vi "Timing Message Loop.vi"(8 "error in (no error)":errorcluster, 10 "Timers":T1, 11 "Message Queues":T2) -> (0 "error out":errorcluster)   [LabVIEW 2017, in "Message Queue.lvlib"]
uses:
  Message Queue.lvlib
  All Message Queues.ctl
  Message Cluster.ctl
  Acquisition/Acquisition State.ctl
  11995cb8-e311-3fce-f8c0-29dfdff9c03f.vi
  controls/ExitGlobal.vi
  Enqueue Message (Single).vi
  <vilib>/Utility/error.llb/Error Cluster From Error Code.vi
  <vilib>/ErrorRing/Error Ring.xnode
  Acquisition/Acquisition.lvlib
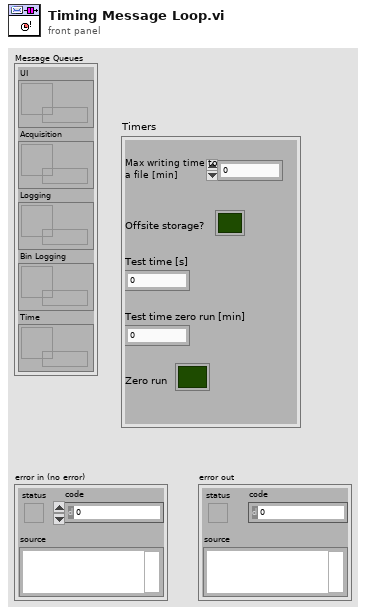
[diagram p1: front panel]
types:
  T1 = cluster{"Offsite storage?":bool, "Test time [s]":dbl, "Test time zero run [s] ":dbl, "Max writing time to a file [min]":dbl, "Zero run":bool}
  T2 = typedef "Message Queue.lvlib/All Message Queues.ctl" = cluster{"UI":refnum<queue>, "Acquisition":refnum<queue>, "Logging":refnum<queue>, "Bin Logging":refnum<queue>, "Time":refnum<queue>}
  T3 = typedef "Acquisition.lvlib/Acquisition State.ctl" = enum16{"Idle", "Acquiring"}
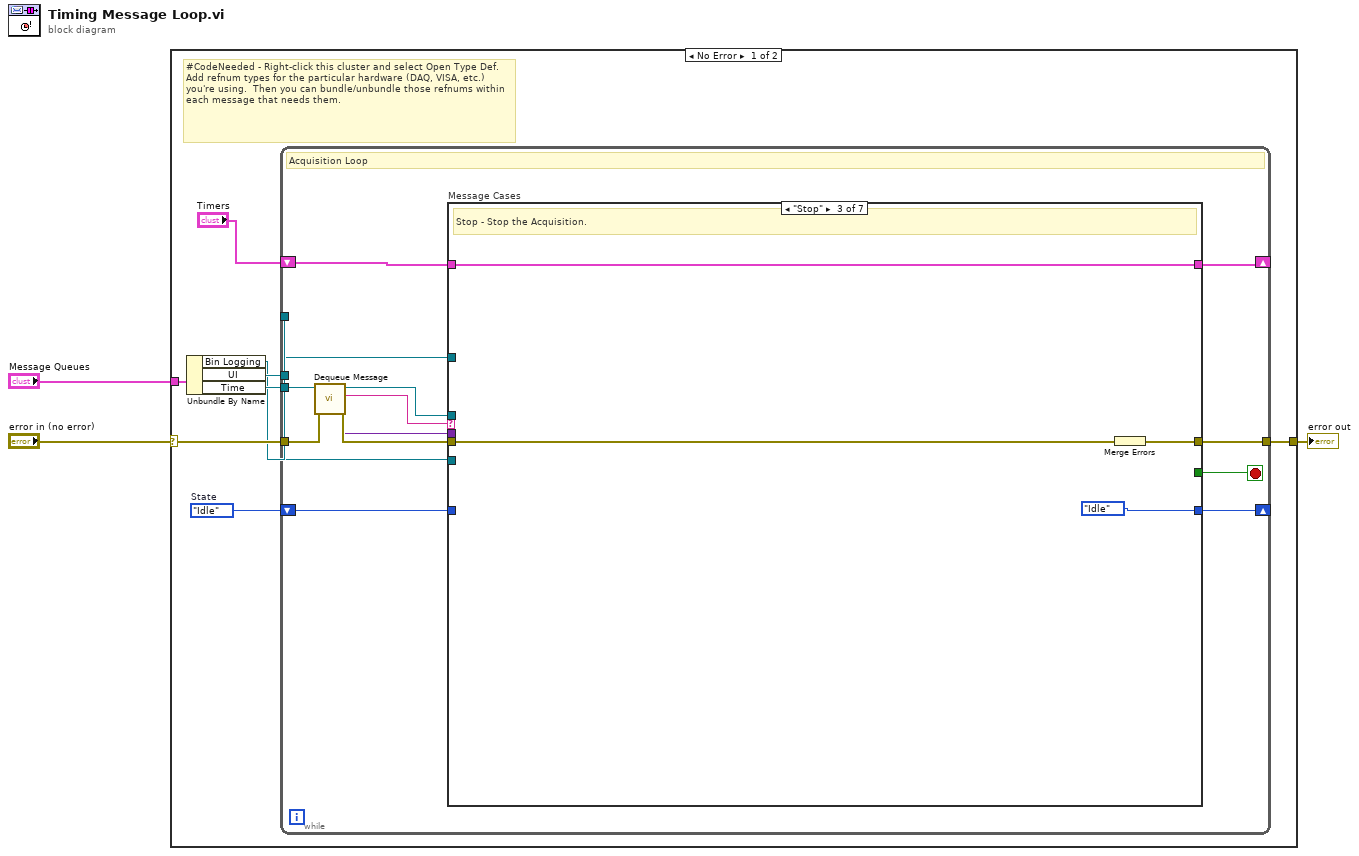
[diagram p0: block diagram]
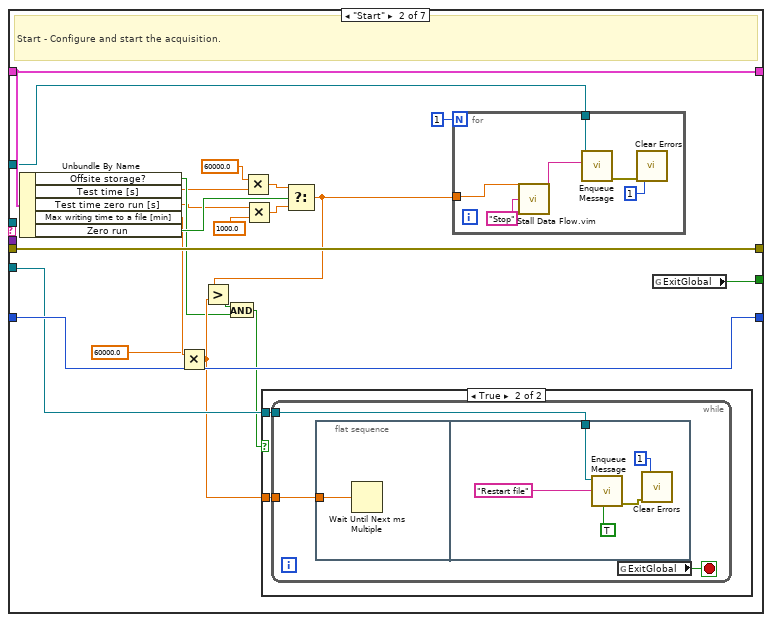
[diagram p3: hidden frame]
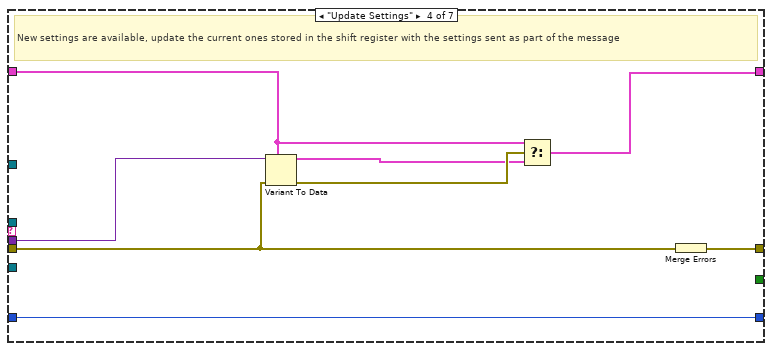
[diagram p5: hidden frame]
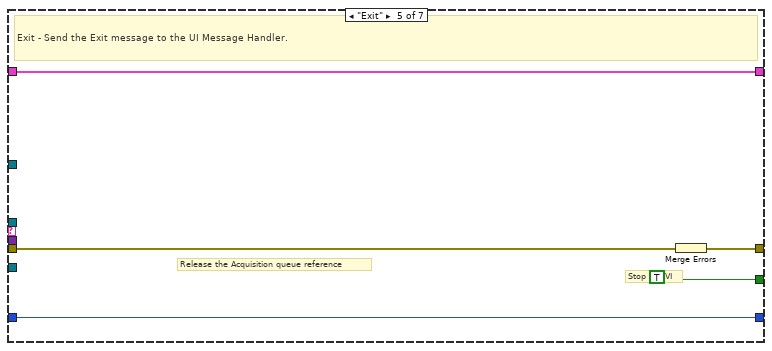
[diagram p6: hidden frame]
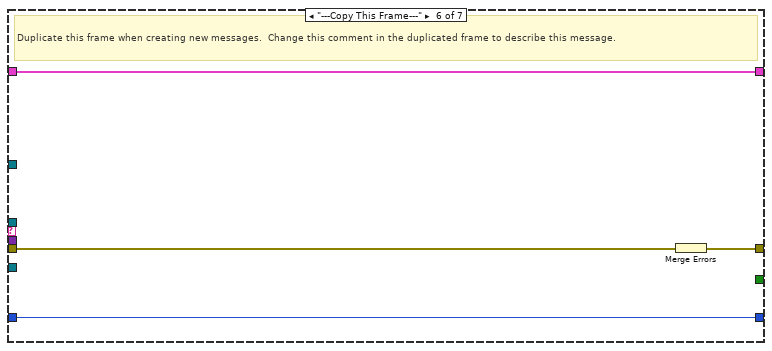
[diagram p7: hidden frame]
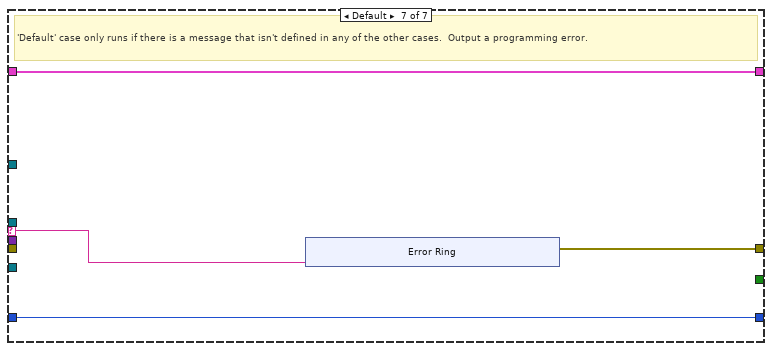
[diagram p8: hidden frame]
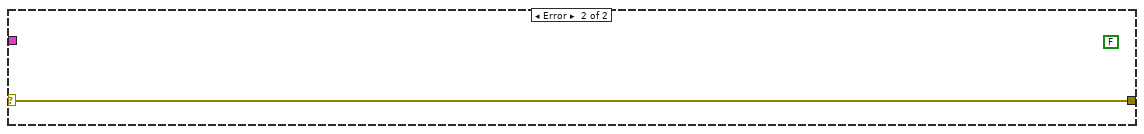
[diagram p9: hidden frame]
diagram:
  n1 = case shown="No Error" "error in (no error)" {
    selector: "error in (no error)" -> [w9 w99]
    tunnel: "Message Queues" -> [w11 _]
    tunnel: [w5 w99] -> w2
    frame No Error {
      w7 = Acquisition_State."Idle"  # State
      # "#CodeNeeded - Right-click this cluster and select Open Type Def.  Add refnum types for the particular hardware (DAQ, VISA, etc.) you're using.  Then you can bundle/unbundle those refnums within each message that needs them."
      n2 = Unbundle By Name(w11) -> ("Bin Logging"=w4:refnum<queue>, "UI"=w8:refnum<queue>, "Time"=w10:refnum<queue>)
      n3 = while {
        tunnel: w10 -> [w20]
        shift-right: [w24] -> _
        shift-left: "Timers" -> [w25]
        tunnel: w8 -> [w16]
        shift-right: [w18] -> _
        shift-left: w7 -> [w19]
        tunnel: w9 -> [w22]
        tunnel: [w15] -> w5
        tunnel: w4 -> [w14]
        stop <- w23 stop-if-true
        # "Acquisition Loop"
        n4 = call "Dequeue Message.vi"("error in (no error)"=w22, "Message Queue"=w20) -> ("error out"=w21:errorcluster, "Message Data"=w13:variant, "Message"=w12:string, "dup Message Queue"=w17:refnum<queue>)  [unwired: 6 in]
        n5 = case "Message Cases" shown="\"Stop\"" w12 {
          selector: w12 -> [_ _ _ _ _ _ w88]
          tunnel: w17 -> [_ _ _ _ _ _ _]
          tunnel: w21 -> [w28 w49 w68 w74 w79 w87 _]
          tunnel: [w28 w49 w70 w78 w82 w85 w89] -> w15
          tunnel: w25 -> [w27 w46 w69 w71 w81 w86 w91]
          tunnel: [w27 w46 w69 w75 w81 w86 w91] -> w24
          tunnel: [_ w45 _ _ TRUE _ _] -> w23
          tunnel: w13 -> [_ _ _ w72 _ _ _]
          tunnel: w16 -> [_ w37 _ _ _ _ _]
          tunnel: w19 -> [w26 w48 _ w73 w80 w84 w90]
          tunnel: [w26 w48 Acquisition_State."Idle" ("State") w73 w80 w84 w90] -> w18
          tunnel: w14 -> [_ w44 _ _ _ _ _]
          frame "Initialize" {
            # "Initialize  - Initialize is currently a no-op.  The hardware initialization takes place in the 'Start' message."
          }
          frame "Start" {
            # "Start - Configure and start the acquisition."
            n6 = Unbundle By Name(w46) -> ("Offsite storage?"=w38:bool, "Test time [s]"=w31:dbl, "Test time zero run [s]"=w35:dbl, "Max writing time to a file [min]"=w43:dbl, "Zero run"=w47:bool)
            n7 = Multiply(x=w43, y=60000.0) -> (x*y=w39:dbl)
            n8 = Multiply(x=60000.0 ("y"), y=w31) -> (x*y=w33:dbl)
            n9 = Multiply(x=w35, y=1000.0) -> (x*y=w32:dbl)
            n10 = Select(t=w33, s=w47, f=w32) -> (s? t:f=w30:dbl)
            n11 = Greater?(x=w30, y=w39) -> (0:w40:bool)
            n12 = And(x=w40, y=w38) -> (x .and. y?=w41:bool)
            n13 = case shown="True" w41 {
              tunnel: w44 -> [_ w57]
              tunnel: w39 -> [_ w56]
              frame False {
              }
              frame True {
                n14 = while {
                  tunnel: w57 -> [w60]
                  tunnel: w56 -> [w59]
                  stop <- w58 stop-if-true
                  n15 = flat-sequence {
                    tunnel: w59 -> [w61]
                    tunnel: w60 -> [w63]
                    frame #0 {
                      n16 = Wait Until Next ms Multiple(millisecond multiple=w61) -> ()  [unwired: 1 out]
                    }
                    frame #1 {
                      n17 = call-poly "Enqueue Message.vi"("Priority Message? (F)"=TRUE, "Message"="Restart file" ("t"), "Message Queue"=w63) -> ("error out"=w66:errorcluster)  [unwired: 7 in, 1 out]
                      n18 = call <vilib>:"Clear Errors.vi"("error in (no error)"=w66, "specific error code to clear (0: all)"=1) -> ()  [unwired: 4 in, 2 out]
                    }
                  }
                  n19 = global read "ExitGlobal.vi" "ExitGlobal"() -> (w58:bool)
                }
              }
            }
            n20 = for {
              N: 1 -> [_]
              tunnel: w37 -> [w51]
              tunnel: w30 -> [w50]
              n21 = call "Stall Data Flow.vim"("value in"="Stop", "milliseconds to wait"=w50) -> ("value out"=w55:string)  [unwired: 1 out]
              n22 = call-poly "Enqueue Message.vi"("Message"=w55, "Message Queue"=w51) -> ("error out"=w52:errorcluster)  [unwired: 8 in, 1 out]
              n23 = call <vilib>:"Clear Errors.vi"("error in (no error)"=w52, "specific error code to clear (0: all)"=1) -> ()  [unwired: 4 in, 2 out]
            }
            n24 = global read "ExitGlobal.vi" "ExitGlobal"() -> (w45:bool)
          }
          frame "Stop" {
            # "Stop - Stop the Acquisition."
            n25 = Merge Errors(w68) -> (w70:errorcluster)
          }
          frame "Update Settings" {
            # "New settings are available, update the current ones stored in the shift register with the settings sent as part of the message"
            n26 = Variant To Data(error in=w74, type=w71, Variant=w72) -> (data=w76:T1, error out=w77:errorcluster)
            n27 = Select(t=w71, s=w77, f=w76) -> (s? t:f=w75:T1)
            n28 = Merge Errors(w74) -> (w78:errorcluster)
          }
          frame "Exit" {
            # "Release the Acquisition queue reference"
            # "Stop the VI"
            # "Exit - Send the Exit message to the UI Message Handler."
            n29 = Merge Errors(w79) -> (w82:errorcluster)
          }
          frame "---Copy This Frame---" {
            # "Duplicate this frame when creating new messages.  Change this comment in the duplicated frame to describe this message."
            n30 = Merge Errors(w87) -> (w85:errorcluster)
          }
          frame Default {
            # "'Default' case only runs if there is a message that isn't defined in any of the other cases.  Output a programming error."
            n31 = xnode "Error Ring"("parameter 0"=w88) -> ("error out"=w89:errorcluster)
          }
        }
      }
    }
    frame Error {
      (unwired) FALSE ("Running")
    }
  }
  "error out" <- w2
